vi "Pockels Cal-Cal subset info-default.vi"(9 "Calibration data array (inc. data header row)":string[][](array[string]), 11 "Cal subset indexes info":string[][](array[string])) -> (2 "Cal subset info array":string[][](array[string]))   [LabVIEW 2020]
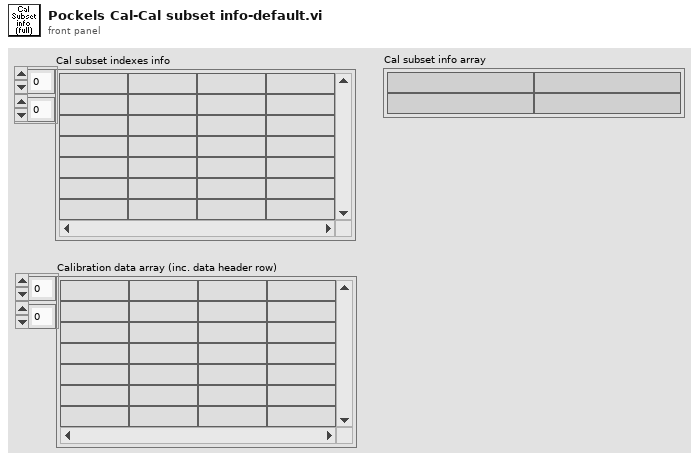
[diagram p1: front panel]
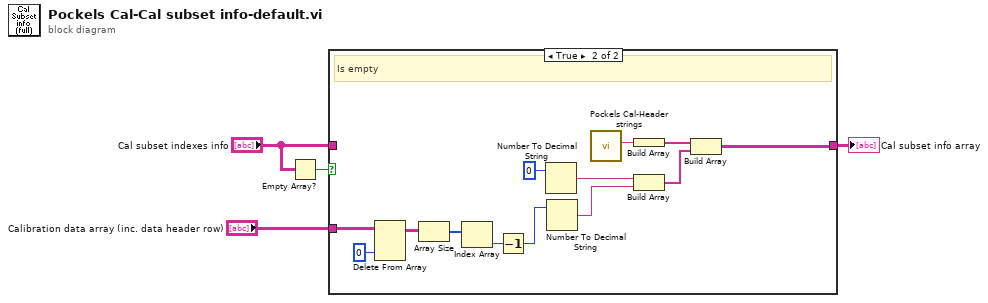
[diagram p0: block diagram]
diagram:
  n1 = Empty Array?(array="Cal subset indexes info") -> (empty?=w3:bool)
  n2 = case shown="True" w3 {
    tunnel: [w5 w14] -> w4
    tunnel: "Cal subset indexes info" -> [w5 _]
    tunnel: "Calibration data array (inc. data header row)" -> [_ w11]
    frame False {
      # "Not empty"
    }
    frame True {
      # "Is empty"
      n3 = Delete From Array(array=w11, index (row)=0) -> (array with subset deleted=w9:string[][])  [unwired: 2 in, 1 out]
      n4 = Array Size(array=w9) -> (size(s)=w8:i32[])
      n5 = Index Array(array=w8) -> (element=w7:i32)  [unwired: 1 in]
      n6 = Decrement(x=w7) -> (x-1=w6:i32)
      n7 = Number To Decimal String(number=0) -> (decimal integer string=w17:string)  [unwired: 1 in]
      n8 = Number To Decimal String(number=w6) -> (decimal integer string=w16:string)  [unwired: 1 in]
      n9 = call "Pockels Cal-Header strings.vi"() -> ("Cal subset indexes header string"=w13:string)  [unwired: 9 in, 2 out]
      n10 = Build Array(w13) -> (w18:string[])
      n11 = Build Array(w17, w16) -> (w15:string[])
      n12 = Build Array(w18, w15) -> (w14:string[][])
    }
  }
  "Cal subset info array" <- w4
